vi "Write ID.vi"(8 "error in (no error)":errorcluster, 10 "ID":u8, 11 "Channel GUI in":refnum<class "Channel GUI.lvclass">) -> (0 "error out":errorcluster, 3 "Channel GUI out":refnum<class "Channel GUI.lvclass">)   [LabVIEW 2018, in "Channel GUI.lvclass"]
uses:
  Channel GUI.lvclass
  Channel GUI.lvclass/Channel GUI.ctl
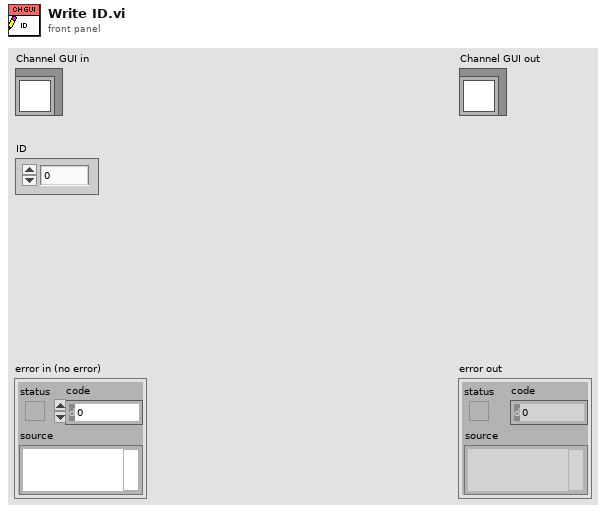
[diagram p1: front panel]
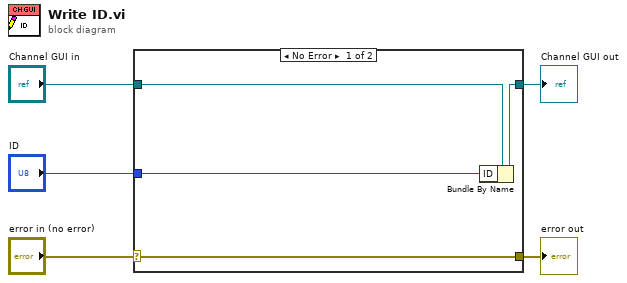
[diagram p0: block diagram]
diagram:
  n1 = case shown="No Error" "error in (no error)" {
    selector: "error in (no error)" -> [w9 w10]
    tunnel: [w9 w10] -> w4
    tunnel: [w7 w11] -> w2
    tunnel: "Channel GUI in" -> [w8 w11]
    tunnel: "ID" -> [w6 _]
    frame No Error {
      n2 = Bundle By Name(cluster=w8, "ID"=w6) -> (w7:refnum<class "Channel GUI.lvclass">)
    }
    frame Error {
    }
  }
  "error out" <- w4
  "Channel GUI out" <- w2
